vi "geve-msg_ui_update_titel_bar.vi"(8 "error in (no error)":errorcluster, 11 "Runtime Data":T1) -> (0 "error out":errorcluster, 3 "Runtime Data out":T1)   [LabVIEW 2018]
doc: "enqueue update title bar action"
uses:
  geve-runtime_data_cluster.ctl
  geve-monitoring_data_cluster.ctl
  geve-serial_config_cluster.ctl
  geve-com_ref_cluster.ctl
  geve-message_cluster.ctl
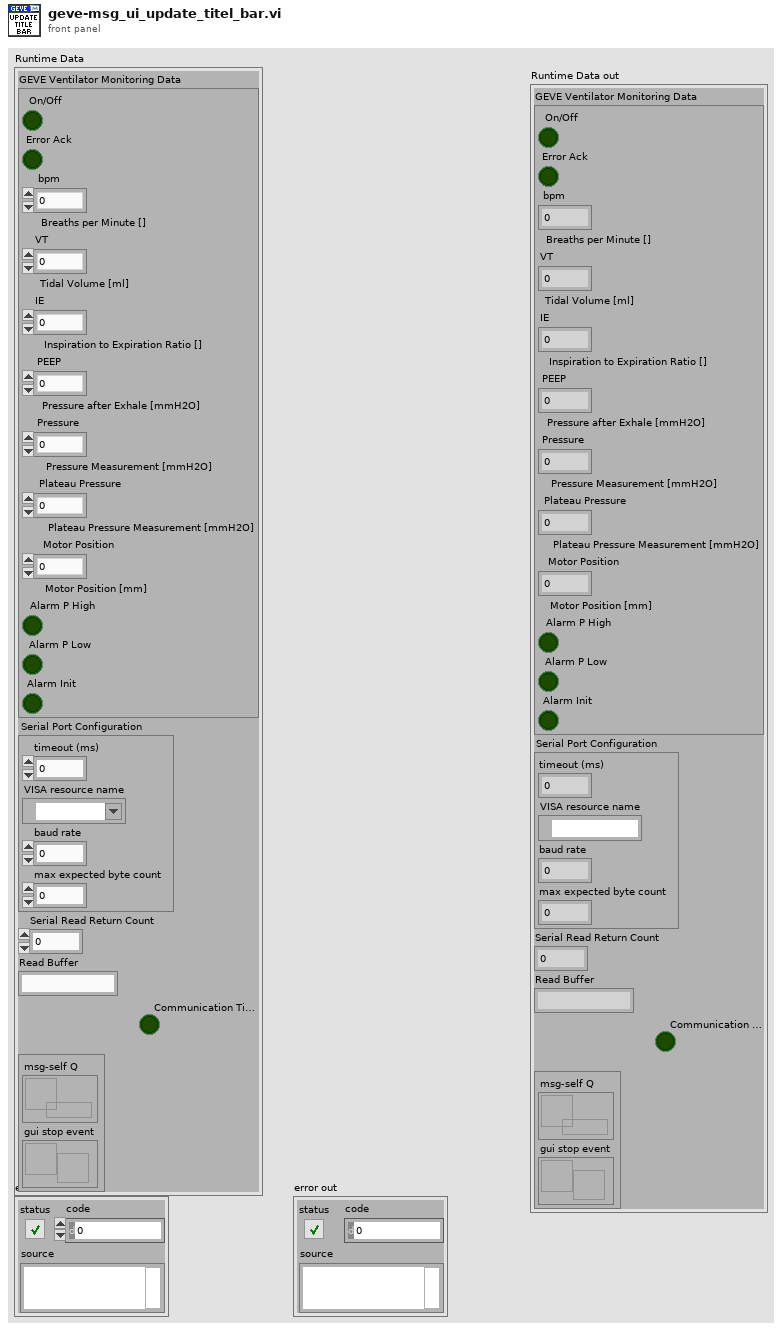
[diagram p1: front panel]
types:
  T1 = typedef "geve-runtime_data_cluster.ctl" = cluster{"GEVE Ventilator Monitoring Data":T2, "Serial Port Configuration":T3, "Serial Read Return Count":u32, "Read Buffer":string, "Communication Timeout?":bool, "com-refs":T4}
  T2 = typedef "geve-monitoring_data_cluster.ctl" = cluster{"On/Off":bool, "Error Ack":bool, "bpm":dbl, "VT":dbl, "IE":dbl, "PEEP":dbl, "Pressure":dbl, "Plateau Pressure":dbl, "Motor Position":dbl, "Alarm P High":bool, "Alarm P Low":bool, "Alarm Init":bool}
  T3 = typedef "geve-serial_config_cluster.ctl" = cluster{"timeout (ms)":u32, "VISA resource name":refnum<visa-resource-name>, "baud rate":u32, "max expected byte count":u32}
  T4 = typedef "geve-com_ref_cluster.ctl" = cluster{"msg-self Q":refnum<queue>, "gui stop event":refnum<user-event>}
  T5 = typedef "geve-message_cluster.ctl" = cluster{"Command":string, "Payload":variant}
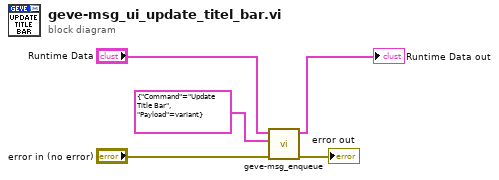
[diagram p0: block diagram]
diagram:
  n1 = call "geve-msg_enqueue.vi"("error in (no error)"="error in (no error)", "Message"=T5 {"Command"="Update Title Bar", "Payload"=variant}, "Runtime Data"="Runtime Data") -> ("error out"=→"error out":errorcluster, "Runtime Data out"=→"Runtime Data out":T1)  [unwired: 7 in]
